vi "host.vi"() -> ()   [LabVIEW 2010]
uses:
  <vilib>/userDefined/High Color/nirio_resource_hc.ctl
  <vilib>/rvi/interface/nirviOpenFPGA/nirviOpenFPGA.xnode
  FPGA Bitfiles/TriggerTest_FPGATarget_main_424F9E99.lvbitx
  <vilib>/rvi/ClientSDK/nirviWhatTheDeviceIsDoing.ctl
  <vilib>/rvi/interface/nirviReadWriteControl/nirviReadWriteControl.xnode
  <vilib>/rvi/interface/common/niFpgaNodeNameForErrorReporting.ctl
  <vilib>/rvi/errors/niLvFpgaWhatHappensToTopLevelVI.ctl
  <vilib>/rvi/interface/nirviMethod/nirviMethod.xnode
  <vilib>/rvi/interface/nirviCloseFPGA/nirviCloseFPGA.xnode
  <vilib>/FPGAPlugInAG/PXI-7813R/niLvFpga_Open_PXI-7813R.vi
  <vilib>/rvi/interface/common/dynamic/niFpgaDynamicAddResources.vi
  <vilib>/Utility/error.llb/Error Cluster From Error Code.vi
  <vilib>/rvi/errors/niLvFpgaAdjustHostInterfaceError.vi
  <vilib>/FPGAPlugInAG/Dynamic/niLvFpga_Reset_Dynamic.vi
  <vilib>/FPGAPlugInAG/Dynamic/niLvFpga_Close_Dynamic.vi
  NiFpgaLv.dll
panel:
  out "Trigger":i16[](graph)
  out "IO 0 36":i16[](graph)
  out "Elements Remaining":u32
  out "FIFO overflow?":bool
  in  "block size":u32=40000
  in  "stop":bool
  out "loop counter":i32
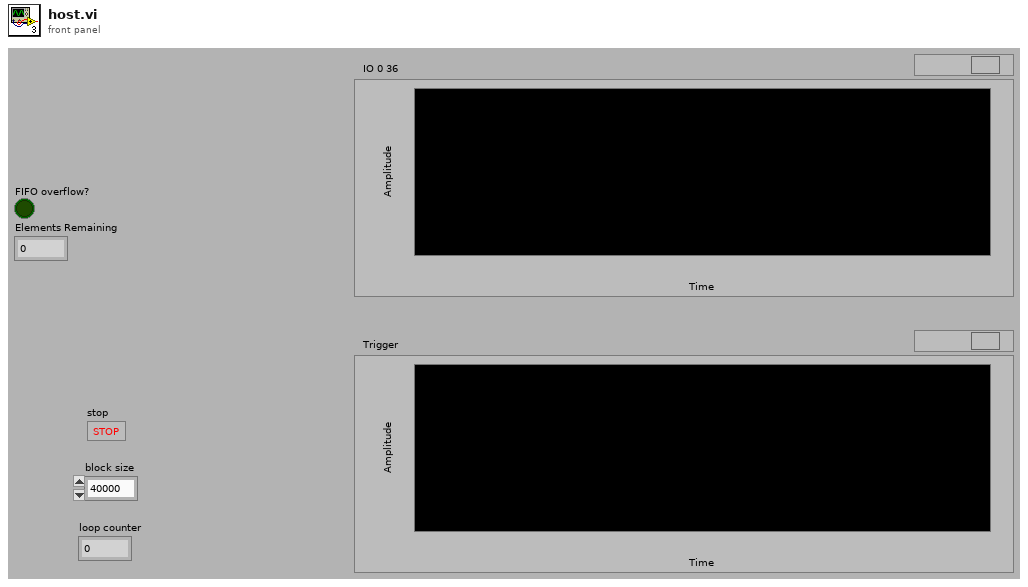
[diagram p1: front panel]
types:
  T1 = typedef "nirio_resource_hc.ctl" = tag
  T2 = typedef "niFpgaNodeNameForErrorReporting.ctl" = enum16{"Open FPGA VI Reference", "Read/Write Control", "Invoke Method: Abort", "Invoke Method: Acknowledge IRQ", "Invoke Method: Download", "Invoke Method: FIFO.Configure", "Invoke Method: FIFO.Read", "Invoke Method: FIFO.Start", "Invoke Method: FIFO.Stop", "Invoke Method: FIFO.Write", "Invoke Method: Reset", "Invoke Method: Run", "Invoke Method: Wait on IRQ", "Close FPGA VI Reference"}
  T3 = typedef "niLvFpgaWhatHappensToTopLevelVI.ctl" = enum16{"top level VI scripted behind XNode", "top level VI inlined behind XNode"}
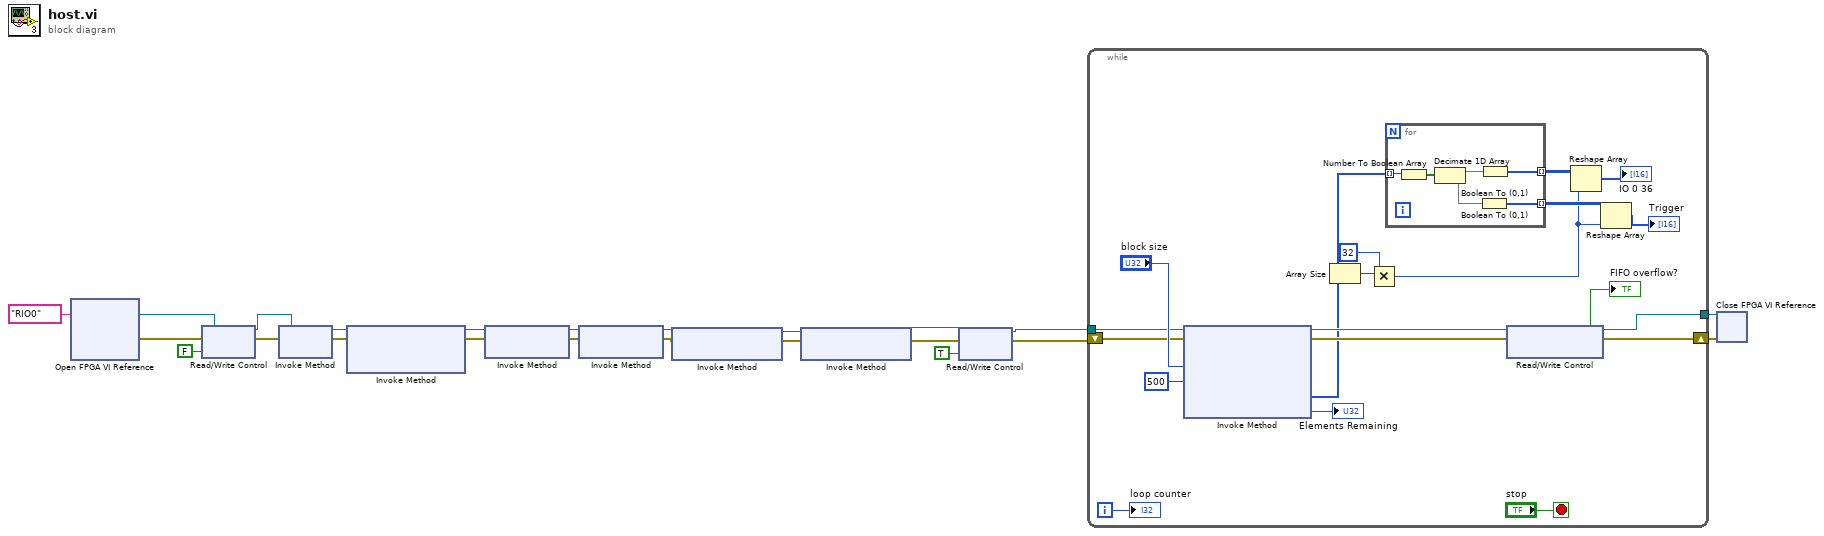
[diagram p0: block diagram]
diagram:
  n1 = xnode "Open FPGA VI Reference"("resource name"=T1 "RIO0") -> ("FPGA VI Reference Out"=w3:refnum<k20>, "error out"=w1:errorcluster)  [unwired: 1 in]
  n2 = xnode "Read/Write Control"("FPGA VI Reference In"=w3, "error in"=w1, "start"=FALSE) -> ("FPGA VI Reference Out"=w2:refnum<k20>, "error out"=w4:errorcluster)
  n3 = xnode "Invoke Method"("FPGA VI Reference In"=w2, "error in"=w4) -> ("FPGA VI Reference Out"=w20:refnum<k20>, "error out"=w19:errorcluster)
  n4 = xnode "Invoke Method"("FPGA VI Reference In"=w20, "error in"=w19) -> ("FPGA VI Reference Out"=w12:refnum<k20>, "error out"=w16:errorcluster)  [unwired: 1 in]
  n5 = xnode "Invoke Method"("FPGA VI Reference In"=w12, "error in"=w16) -> ("FPGA VI Reference Out"=w18:refnum<k20>, "error out"=w17:errorcluster)
  n6 = xnode "Invoke Method"("FPGA VI Reference In"=w18, "error in"=w17) -> ("FPGA VI Reference Out"=w11:refnum<k20>, "error out"=w13:errorcluster)
  n7 = xnode "Invoke Method"("FPGA VI Reference In"=w11, "error in"=w13) -> ("FPGA VI Reference Out"=w14:refnum<k20>, "error out"=w15:errorcluster)
  n8 = xnode "Invoke Method"("FPGA VI Reference In"=w14, "error in"=w15) -> ("FPGA VI Reference Out"=w8:refnum<k20>, "error out"=w6:errorcluster)
  n9 = xnode "Read/Write Control"("FPGA VI Reference In"=w8, "error in"=w6, "start"=TRUE) -> ("FPGA VI Reference Out"=w7:refnum<k20>, "error out"=w9:errorcluster)
  n10 = while {
    shift-right: [w37] -> w23
    shift-left: w9 -> [w35]
    tunnel: [w39] -> w22
    tunnel: w7 -> [w34]
    i -> [w43]
    stop <- "stop" stop-if-true
    n11 = xnode "Invoke Method"("FPGA VI Reference In"=w34, "error in"=w35, "Number of Elements"="block size", "Timeout (ms)"=500) -> ("FPGA VI Reference Out"=w40:refnum<k20>, "error out"=w38:errorcluster, "Data"=w30:u64[], "Elements Remaining"=→"Elements Remaining":u32)
    n12 = Array Size(array=w30) -> (size(s)=w29:i32)
    n13 = Multiply(x=w29, y=32) -> (x*y=w25:i32)
    n14 = for {
      tunnel: w30 -> [w49] mode=indexing
      tunnel: [w46] -> w31 mode=indexing
      tunnel: [w44] -> w26 mode=indexing
      n15 = Number To Boolean Array(number=w49) -> (Boolean array=w48:bool[])
      n16 = Decimate 1D Array(w48) -> (w47:bool[], w45:bool[])
      n17 = Boolean To (0,1)(Boolean=w45) -> (0, 1=w44:i16[])
      n18 = Boolean To (0,1)(Boolean=w47) -> (0, 1=w46:i16[])
    }
    n19 = xnode "Read/Write Control"("FPGA VI Reference In"=w40, "error in"=w38) -> ("FPGA VI Reference Out"=w39:refnum<k20>, "error out"=w37:errorcluster, "FIFO overflow?"=→"FIFO overflow?":bool)
    n20 = Reshape Array(w31, w25) -> (→"IO 0 36":i16[])
    n21 = Reshape Array(w26, w25) -> (→"Trigger":i16[])
    "loop counter" <- w43
  }
  n22 = xnode "Close FPGA VI Reference"("FPGA VI Reference In"=w22, "error in"=w23) -> ()  [unwired: 1 out]
